vi "readProductDataInProductTable.vi"(8 "error in":errorcluster, 11 "dataToQueryOfRead":T1) -> (0 "error out":errorcluster, 3 "ClusterFormat":T1)   [LabVIEW 2014]
uses:
  <vilib>/addons/database/Connection.llb/DB Tools Open Connec (String).vi
  <vilib>/addons/database/Auxilliary.llb/DB Tools Format Datetime String (Time Stamp).vi
  <vilib>/addons/database/NI_Database_API.lvlib
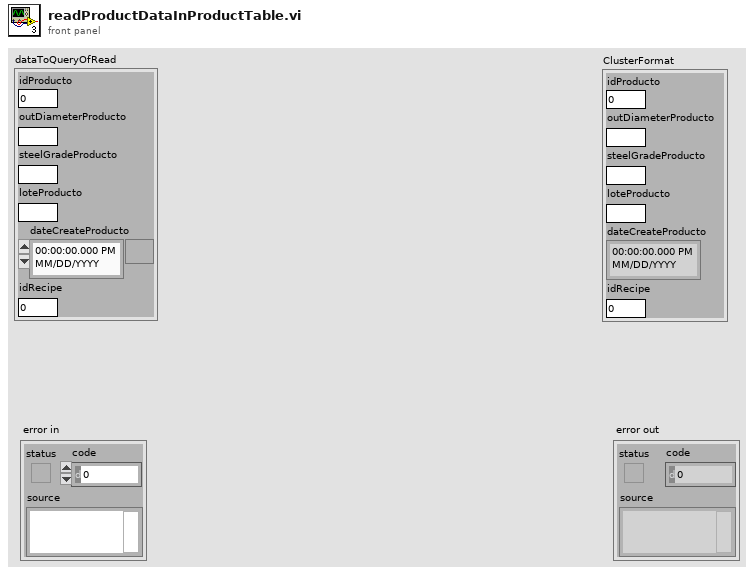
[diagram p1: front panel]
types:
  T1 = cluster{"idProducto":dbl, "outDiameterProducto":string, "steelGradeProducto":string, "loteProducto":string, "dateCreateProducto":timestamp, "idRecipe":dbl}
  T2 = typedef "NI_Database_API.lvlib/Conn ObjectReference.ctl" = refnum<k1>
  T3 = typedef "NI_Database_API.lvlib/DB Tools DataTypes.ctl" = enum16{"String", "Long (I32)", "Single (SGL)", "Double (DBL)", "Date/Time", "Binary"}
  T4 = cluster{"name":string, "database data type":T3, "defined size":i32}[]
  T5 = cluster{string, "outDiameterProducto":string, "steelGradeProducto":string, "loteProducto":string, "date/time string":string, string}
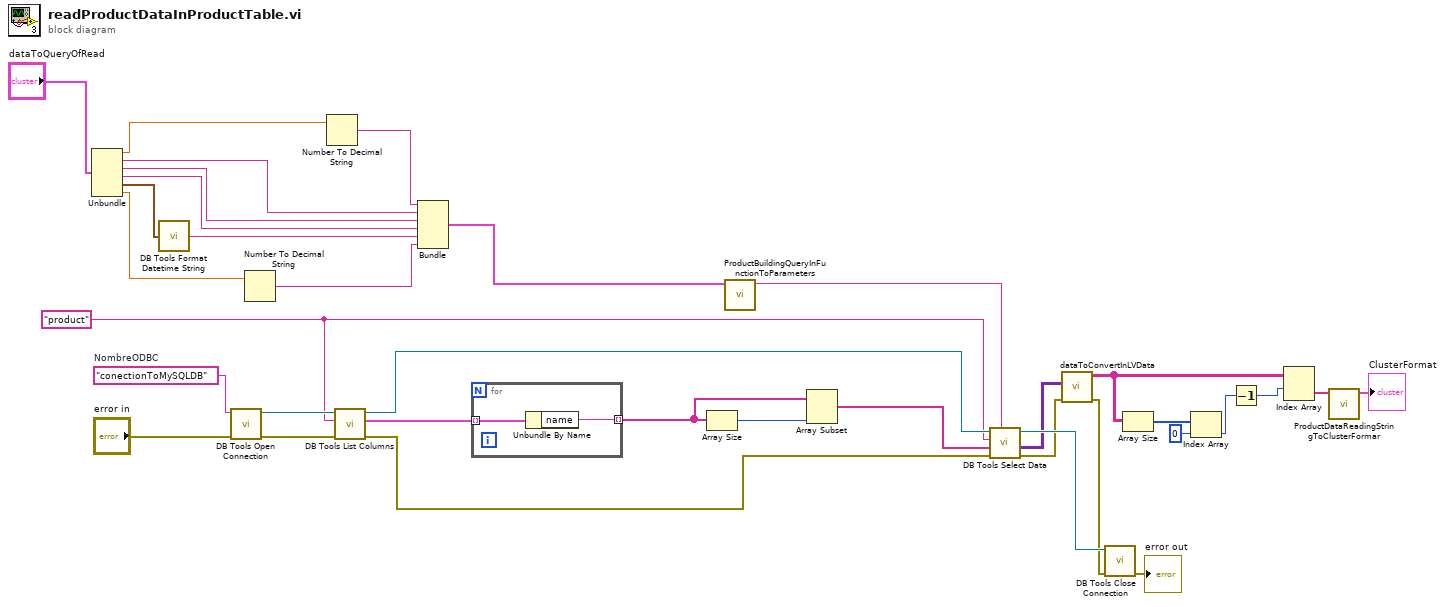
[diagram p0: block diagram]
diagram:
  w22 = "product" ("tableName")
  w35 = "conectionToMySQLDB"  # NombreODBC
  n1 = Unbundle("dataToQueryOfRead") -> ("idProducto"=w29:dbl, "outDiameterProducto"=w28:string, "steelGradeProducto"=w12:string, "loteProducto"=w11:string, "dateCreateProducto"=w13:timestamp, "idRecipe"=w9:dbl)
  n2 = call-poly <vilib>:"DB Tools Format Datetime String.vi"("time stamp"=w13) -> ("date/time string"=w10:string)
  n3 = call-poly <vilib>:"DB Tools Open Connection.vi"("error in (no error)"="error in", "connection information"=w35) -> ("error out"=w33:errorcluster, "connection reference"=w34:T2)  [unwired: 6 in]
  n4 = Number To Decimal String(number=w9) -> (decimal integer string=w8:string)  [unwired: 1 in]
  n5 = Number To Decimal String(number=w29) -> (decimal integer string=w30:string)  [unwired: 1 in]
  n6 = call <vilib>:"DB Tools List Columns.vi"("error in (no error)"=w33, "table"=w22, "connection reference"=w34) -> ("error out"=w23:errorcluster, "column information"=w31:T4, "connection reference out"=w24:T2)  [unwired: 1 in, 1 out]
  n7 = Bundle(w30, "outDiameterProducto"=w28, "steelGradeProducto"=w12, "loteProducto"=w11, "date/time string"=w10, w8) -> (w6:T5)  [unwired: 1 in]
  n8 = for {
    tunnel: w31 -> [w37] mode=indexing
    tunnel: [w36] -> w26 mode=indexing
    n9 = Unbundle By Name(w37) -> ("name"=w36:string)
  }
  n10 = Array Size(array=w26) -> (size(s)=w27:i32)
  n11 = call "ProductBuildingQueryInFunctionToParameters.vi"("ParameterToRead"=w6) -> ("QueryToRead"=w21:string)  [unwired: 10 in]
  n12 = Array Subset(array=w26, length=w27) -> (w25:string[])  [unwired: 1 in]
  n13 = call <vilib>:"DB Tools Select Data.vi"("condition"=w21, "error in (no error)"=w23, "columns"=w25, "table"=w22, "connection reference"=w24) -> ("error out"=w17:errorcluster, "data"=w18:variant[][], "connection reference out"=w20:T2)  [unwired: 1 in]
  n14 = call "dataToConvertInLVData.vi"("error in"=w17, "dataReadingIn"=w18) -> ("error out"=w16:errorcluster, "dataReadingOut"=w2:string[][])  [unwired: 8 in]
  n15 = call <vilib>:"DB Tools Close Connection.vi"("error in (no error)"=w16, "connection reference"=w20) -> ("error out"=→"error out":errorcluster)  [unwired: 5 in]
  n16 = Array Size(array=w2) -> (size(s)=w5:i32[])
  n17 = Index Array(array=w5, index=0) -> (element=w3:i32)
  n18 = Decrement(x=w3) -> (x-1=w1:i32)
  n19 = Index Array(array=w2, index (row)=w1) -> (element=w15:string[])  [unwired: 1 in]
  n20 = call "ProductDataReadingStringToClusterFormar.vi"("StringFormat"=w15) -> ("ClusterFormat"=→"ClusterFormat":T1)  [unwired: 10 in]
